vi "OSP.vi"() -> ()   [LabVIEW 2019]
uses:
  <vilib>/vision/NI_Vision_Development_Module.lvlib
panel:
  out "Image":T1(plugin-control)
  out "return value 3":i32[](array[numeric])
  in  "Path Control":path
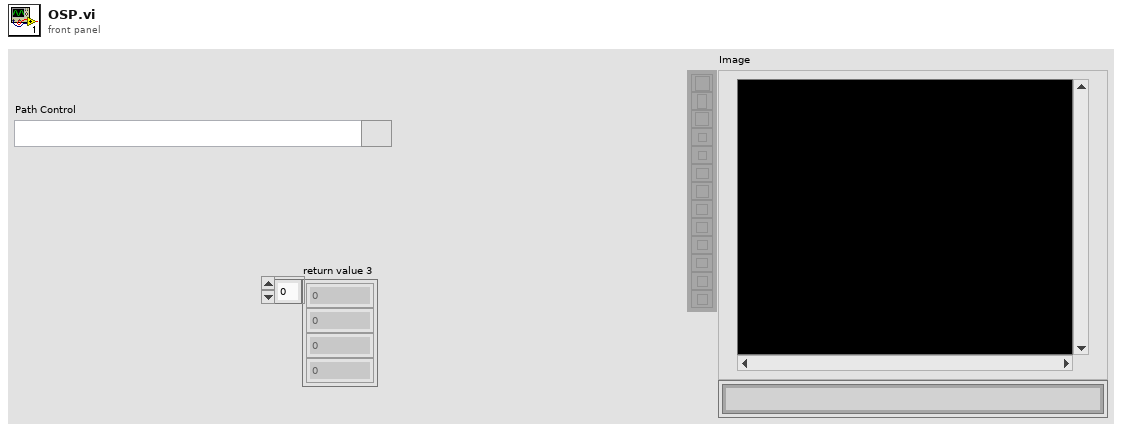
[diagram p1: front panel]
types:
  T1 = typedef "IMAQ Image.ctl" = refnum<image>
  T2 = typedef "Image Type" = u32
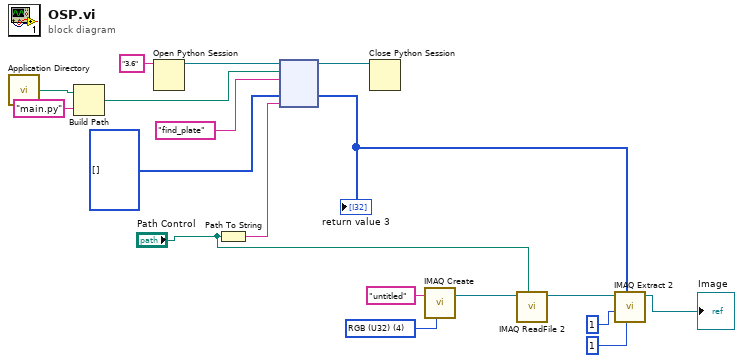
[diagram p0: block diagram]
diagram:
  w8 = T2 4 items=["Grayscale (U8)", "Grayscale (I16)", "Grayscale (SGL)", "Complex (CSG)", "RGB (U32)", "HSL (U32)", "RGB (U64)", "Grayscale (U16)"] ("Image Type")
  n1 = call <vilib>:"Application Directory.vi"() -> ("Application Directory"=w12:path)
  n2 = Build Path(base path=w12, name or relative path="main.py") -> (appended path=w10:path)
  n3 = Open Python Session(python version="3.6" ("Python version")) -> (session out=w17:refnum<k35>)  [unwired: 2 in, 1 out]
  n4 = Path To String(path="Path Control") -> (string=w14:string)
  n5 = node(w17, w10, "find_plate" ("function name"), i32[] [], w14) -> (w16:refnum<k35>, w1:i32[])  [unwired: 2 in, 3 out]
  "return value 3" <- w1
  n6 = Close Python Session(session in=w16) -> ()  [unwired: 1 in, 1 out]
  n7 = call "IMAQ Create"("Image Name"="untitled", "Image Type"=w8) -> ("New Image"=w7:T1)  [unwired: 3 in, 1 out]
  n8 = call "IMAQ ReadFile 2"("File Path"="Path Control", "Image"=w7) -> ("Image Out"=w5:T1)  [unwired: 5 in, 4 out]
  n9 = call "IMAQ Extract 2"("Y Step Size"=1, "Optional Rectangle"=w1, "X Step Size"=1, "Image Src"=w5) -> ("Image Dst Out"=→"Image":T1)  [unwired: 6 in, 1 out]
